vi "AdvancedCurveFit.vi"(8 "error in (no error)":errorcluster, 9 "initial guess coefficients":dbl[](array[numeric])=[0.0, 0.0, 0.0, 0.0, 0.0], 10 "Locations":dynamicdata(graph), 11 "Signals":dynamicdata(graph)) -> (0 "error out":errorcluster, 1 "mean squared error":dynamicdata(graph), 2 "residual":dynamicdata(graph), 3 "best fit":dynamicdata(graph), 4 "non-linear coefficients":dynamicdata(graph))   [LabVIEW 2020]
doc: "Computes the coefficients that best represent the input data based on the chosen model type.\n--------------------\n\nThis Express VI is configured as follows:\n\nModel type: Non-linear\nModel description: v*s+i-a*exp(abs(v0+v)*c)\nIndependent variable: v\nMaximum iterations: 500"
panel:
  in  "Tab Control 2":enum32{"Signals In", "Signals In 2"}(tab)
  out "Signals In":dynamicdata(graph)
  out "Signals In 2":dynamicdata(graph)
  in  "Tab Control":T1(tab)
  out "slope":dynamicdata(graph)
  out "intercept":dynamicdata(graph)
  out "a0":dynamicdata(graph)
  out "a1":dynamicdata(graph)
  out "a2":dynamicdata(graph)
  out "polynomial coefficients":dynamicdata(graph)
  out "spline interpolant":dynamicdata(graph)
  out "general LS coefficients":dynamicdata(graph)
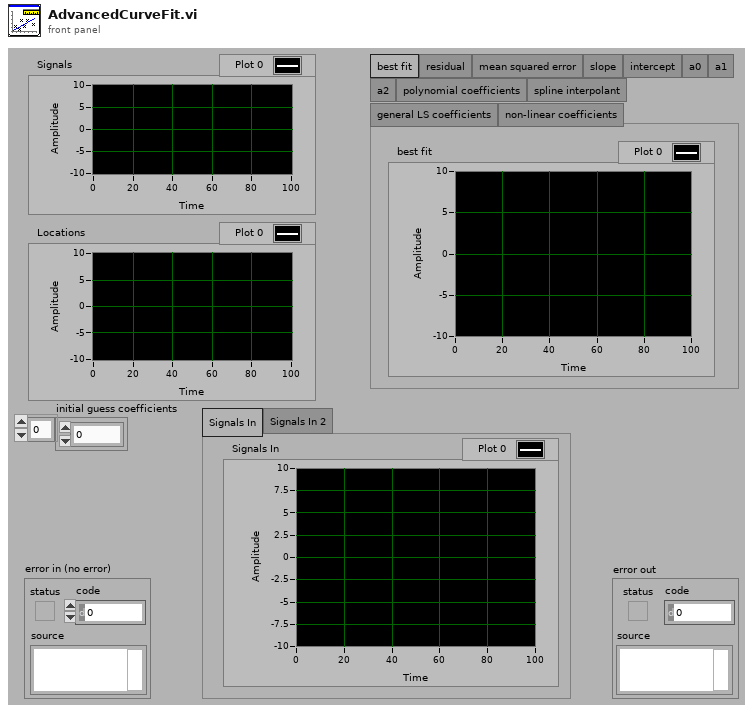
[diagram p1: front panel]
types:
  T1 = enum32{"best fit", "residual", "mean squared error", "slope", "intercept", "a0", "a1", "a2", "polynomial coefficients", "spline interpolant", "general LS coefficients", "non-linear coefficients"}
  T2 = enum16{"Linear", "Quadratic", "Cubic Spline", "Polynomial", "General LS Linear", "Non-Linear"}
  T3 = cluster{"model":string, "Parameters":string[], "x":string}
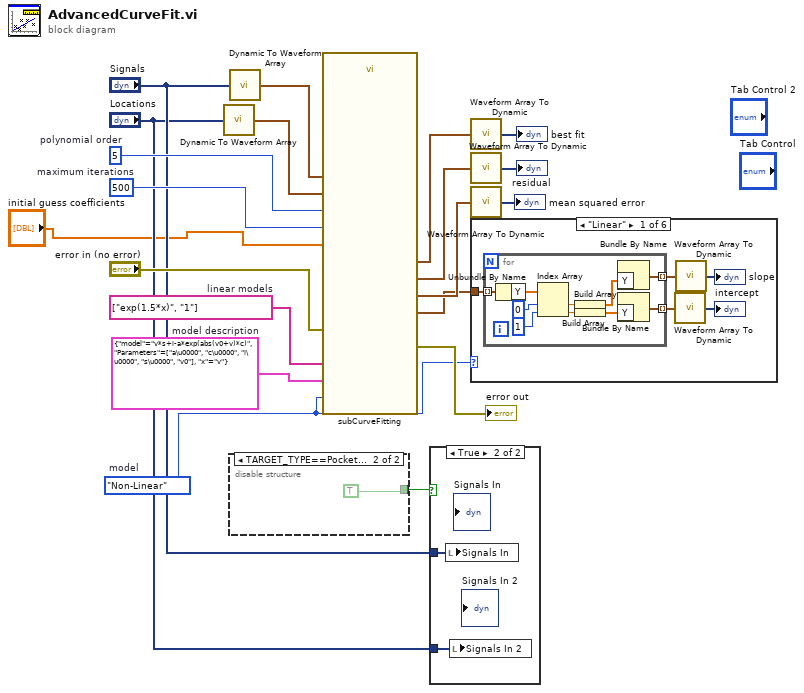
[diagram p0: block diagram]
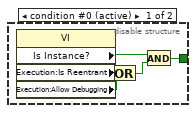
[diagram p2: hidden frame]
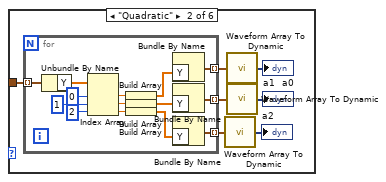
[diagram p4: hidden frame]
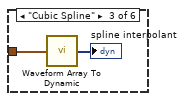
[diagram p5: hidden frame]
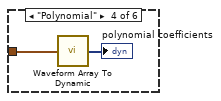
[diagram p6: hidden frame]
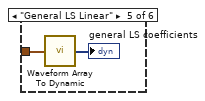
[diagram p7: hidden frame]
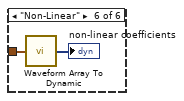
[diagram p8: hidden frame]
diagram:
  w12 = T2."Non-Linear"  # model
  w8 = T3 {"model"="v*s+i-a*exp(abs(v0+v)*c)", "Parameters"=["a\u0000", "c\u0000", "i\u0000", "s\u0000", "v0"], "x"="v"}  # model description
  w9 = string[] ["exp(1.5*x)", "1"]  # linear models
  w19 = 5  # polynomial order
  w13 = 500  # maximum iterations
  n1 = call <vilib>:"Dynamic To Waveform Array.vi"("Input"="Locations") -> ("Output"=w5:waveform(dbl)[])  [unwired: 4 in]
  n2 = call <vilib>:"Dynamic To Waveform Array.vi"("Input"="Signals") -> ("Output"=w20:waveform(dbl)[])  [unwired: 4 in]
  n3 = disable-structure shown="TARGET_TYPE==PocketPC||TARGET_TYPE==PalmOS||TARGET_TYPE==Embedded" {
    disable-tunnel: [w21 TRUE] -> w2
    frame condition #0 (active) {
      n4 = property class="VI"() -> ("Is Instance?"=w25:bool, "Execution:Is Reentrant"=w23:bool, "Execution:Allow Debugging"=w22:bool)  [unwired: 2 in, 2 out]
      n5 = Or(x=w23, y=w22) -> (x .or. y?=w24:bool)
      n6 = And(x=w25, y=w24) -> (x .and. y?=w21:bool)
    }
    frame condition #1 {
    }
  }
  n7 = call <vilib>:"subCurveFitting.vi"("signals"=w20, "model description"=w8, "Initial Guess Coefficient"="initial guess coefficients", "locations"=w5, "model"=w12, "polynomial order"=w19, "error in"="error in (no error)", "linear models"=w9, "max iteration"=w13) -> ("best fit"=w15:waveform(dbl)[], "residual"=w16:waveform(dbl)[], "best fit coefficients"=w10:waveform(dbl)[], "mse"=w11:waveform(dbl)[], "error out"=→"error out":errorcluster)  [unwired: 2 in]
  n8 = case shown="True" w2 {
    tunnel: "Signals" -> [_ w28]
    tunnel: "Locations" -> [_ w27]
    frame False {
    }
    frame True {
      n9 = local write "Signals In"(w28) -> ()
      n10 = local write "Signals In 2"(w27) -> ()
    }
  }
  n11 = call <vilib>:"Waveform Array To Dynamic.vi"("Input"=w15) -> ("Output"=→"best fit":dynamicdata)  [unwired: 4 in]
  n12 = call <vilib>:"Waveform Array To Dynamic.vi"("Input"=w16) -> ("Output"=→"residual":dynamicdata)  [unwired: 4 in]
  n13 = call <vilib>:"Waveform Array To Dynamic.vi"("Input"=w11) -> ("Output"=→"mean squared error":dynamicdata)  [unwired: 4 in]
  n14 = case shown="\"Linear\"" w12 {
    tunnel: w10 -> [w33 w50 w65 w68 w70 w72]
    frame "Linear" {
      n15 = for {
        tunnel: w33 -> [w43] mode=indexing
        tunnel: [w35] -> w29 mode=indexing
        tunnel: [w34] -> w30 mode=indexing
        n16 = Unbundle By Name(w43) -> ("Y"=w42:dbl[])
        n17 = Index Array(array=w42, index #1=0 ("index"), index #2=1 ("index")) -> (element #1=w38:dbl, element #2=w39:dbl)
        n18 = Build Array(w38) -> (w36:dbl[])
        n19 = Build Array(w39) -> (w37:dbl[])
        n20 = Bundle By Name("Y"=w36) -> (w34:waveform(dbl))  [unwired: 1 in]
        n21 = Bundle By Name("Y"=w37) -> (w35:waveform(dbl))  [unwired: 1 in]
      }
      n22 = call <vilib>:"Waveform Array To Dynamic.vi"("Input"=w29) -> ("Output"=→"intercept":dynamicdata)  [unwired: 4 in]
      n23 = call <vilib>:"Waveform Array To Dynamic.vi"("Input"=w30) -> ("Output"=→"slope":dynamicdata)  [unwired: 4 in]
    }
    frame "Quadratic" {
      n24 = for {
        tunnel: w50 -> [w64] mode=indexing
        tunnel: [w53] -> w44 mode=indexing
        tunnel: [w52] -> w45 mode=indexing
        tunnel: [w51] -> w46 mode=indexing
        n25 = Unbundle By Name(w64) -> ("Y"=w63:dbl[])
        n26 = Index Array(array=w63, index #1=0 ("index"), index #2=1 ("index"), index #3=2 ("index")) -> (element #1=w57:dbl, element #2=w58:dbl, element #3=w59:dbl)
        n27 = Build Array(w57) -> (w54:dbl[])
        n28 = Build Array(w58) -> (w55:dbl[])
        n29 = Build Array(w59) -> (w56:dbl[])
        n30 = Bundle By Name("Y"=w54) -> (w51:waveform(dbl))  [unwired: 1 in]
        n31 = Bundle By Name("Y"=w55) -> (w52:waveform(dbl))  [unwired: 1 in]
        n32 = Bundle By Name("Y"=w56) -> (w53:waveform(dbl))  [unwired: 1 in]
      }
      n33 = call <vilib>:"Waveform Array To Dynamic.vi"("Input"=w44) -> ("Output"=→"a2":dynamicdata)  [unwired: 4 in]
      n34 = call <vilib>:"Waveform Array To Dynamic.vi"("Input"=w46) -> ("Output"=→"a0":dynamicdata)  [unwired: 4 in]
      n35 = call <vilib>:"Waveform Array To Dynamic.vi"("Input"=w45) -> ("Output"=→"a1":dynamicdata)  [unwired: 4 in]
    }
    frame "Cubic Spline" {
      n36 = call <vilib>:"Waveform Array To Dynamic.vi"("Input"=w65) -> ("Output"=→"spline interpolant":dynamicdata)  [unwired: 4 in]
    }
    frame "Polynomial" {
      n37 = call <vilib>:"Waveform Array To Dynamic.vi"("Input"=w68) -> ("Output"=→"polynomial coefficients":dynamicdata)  [unwired: 4 in]
    }
    frame "General LS Linear" {
      n38 = call <vilib>:"Waveform Array To Dynamic.vi"("Input"=w70) -> ("Output"=→"general LS coefficients":dynamicdata)  [unwired: 4 in]
    }
    frame "Non-Linear" {
      n39 = call <vilib>:"Waveform Array To Dynamic.vi"("Input"=w72) -> ("Output"=→"non-linear coefficients":dynamicdata)  [unwired: 4 in]
    }
  }
